vi "interfejs.vi"() -> ()   [LabVIEW 2017]
uses:
  <vilib>/event_ctls.llb/lveventtype.ctl
  <vilib>/Instr/_visa.llb/VISA Configure Serial Port (Instr).vi
  <vilib>/imath/engines/lvmath2/RunTimeEngine/BuiltInFunctions/deg_to_rad/NIMS_deg_to_rad.vi
  <instcachedir>/0/NIMS_deg_to_rad_4A81D684CE8D4DD79924F5AB74D756E1.lvgen/NIMS_deg_to_rad_4A81D684CE8D4DD79924F5AB74D756E1_001.vi
  <vilib>/imath/engines/lvmath2/RunTimeEngine/ArithmeticOperatorToken/NIMS_ArithmeticOperator_multmx-internal.vi
  <instcachedir>/0/NIMS_ArithmeticOperator_multmx-internal_D14B0E8358F948B18FBB33DB0D4CACE1.lvgen/NIMS_ArithmeticOperator_multmx-internal_D14B0E8358F948B18FBB33DB0D4CACE1_004.vi
  <vilib>/imath/engines/lvmath2/RunTimeEngine/ErrorHandling/NIMS_Create Error From Enums.vi
  <vilib>/imath/engines/lvmath2/RunTimeEngine/NodeEndStatement/NIMS_NodeEndStatement_Output.vi
  <instcachedir>/0/NIMS_NodeEndStatement_Output_53EC0D466D134D7ABD903AC30B43404B.lvgen/NIMS_NodeEndStatement_Output_53EC0D466D134D7ABD903AC30B43404B_001.vi
  <vilib>/imath/engines/lvmath2/RunTimeEngine/ErrorHandling/NIMS_Finalize Error.vi
panel:
  out "x/y 5":dbl
  out "x/y 4":dbl
  out "x/y 3":dbl
  out "x/y 2":dbl
  out "x/y":dbl
  in  "SterowanieManipulator":bool
  out "Napięcie akumulatorów":dbl
  out "Temperatura":dbl
  out "Położenie osi skrętnej":u16(knob) scale=0.0..99.0
  out "Zabezpieczenie wyłączenie PWM":string
  out "Kierunek skrętu(1-prawo, 2-lewo)":string
  out "Kierunek jazdy(0-postój, 1-do przodu, 2-do tyłu)":string
  out "readBuffor":string
  out "palec2":i32
  out "pale3":i32
  out "palec4":i32
  out "palec5":i32
  out "X_rekawica":i32
  out "Y_rekawica":i32
  out "palec1":i32
  in  "StartReading":bool
  in  "VISA resource name":refnum<visa-resource-name>
  out "pozycjaSP_manipulator":dbl
  out "pozycjaS1_manipulator":dbl
  out "pozycjaS2_manipulator":dbl
  out "pozycjaS3_manipulator":dbl
  out "Px":dbl
  out "Py":dbl
  out "Pz":dbl
  out "pozycjaS4_manipulator":dbl
  out "pozycjaSn_manipulator":dbl
  in  "UruchomManipulator":bool
  in  "Xn [mm]":dbl=165.0 format="%#_13g"
  in  "X4 [mm]":dbl=205.0 format="%#_13g"
  in  "X3 [mm]":dbl=310.0 format="%#_13g"
  in  "X2[mm]":dbl=400.0 format="%#_13g"
  in  "X1[mm]":dbl=65.0 format="%#_13g"
  in  "Zp [mm]":dbl=465.0 format="%#_13g"
  in  "positionSP [stopnie]":dbl(slide) scale=-85.0..85.0
  in  "positionS1 [stopnie]":dbl(slide)=76.9090909090909 scale=-85.0..85.0
  in  "positionS2 [stopnie]":dbl(slide)=-85.0 scale=-85.0..85.0
  in  "positionS3 [stopnie]":dbl(slide)=-85.0 scale=-85.0..85.0
  in  "positionS4 [stopnie]":dbl(slide)=-52.69090909090909 scale=-85.0..85.0
  in  "positionSn [stopnie]":dbl(slide) scale=-85.0..85.0
  out "ResetPWM_platforma":i16
  out "Brzeczyk_platforma":i16
  out "Swiatla_platforma":i16
  out "BlokadaNapedow_platforma":i16
  out "X_platforma":dbl
  out "Y_platforma":dbl
  out "palce":string
  in  "Typ Sterowania Platforma":bool
  in  "Reset\nzabezpieczenia PWM":bool
  in  "Brzęczyk":bool
  in  "Światła":bool
  in  "Blokada napedów":bool=TRUE
  out "Zadana prędkość":dbl(slide) scale=0.0..99.0
  out "zadany skręt":dbl(slide) scale=0.0..99.0
  out "x1":dbl
  out "y 2":dbl
  in  "Stop":bool
  out "YMysz":dbl
  out "XMysz":dbl
  out "2D Picture":picture
  # "T-rękawica\nF-suwaki"
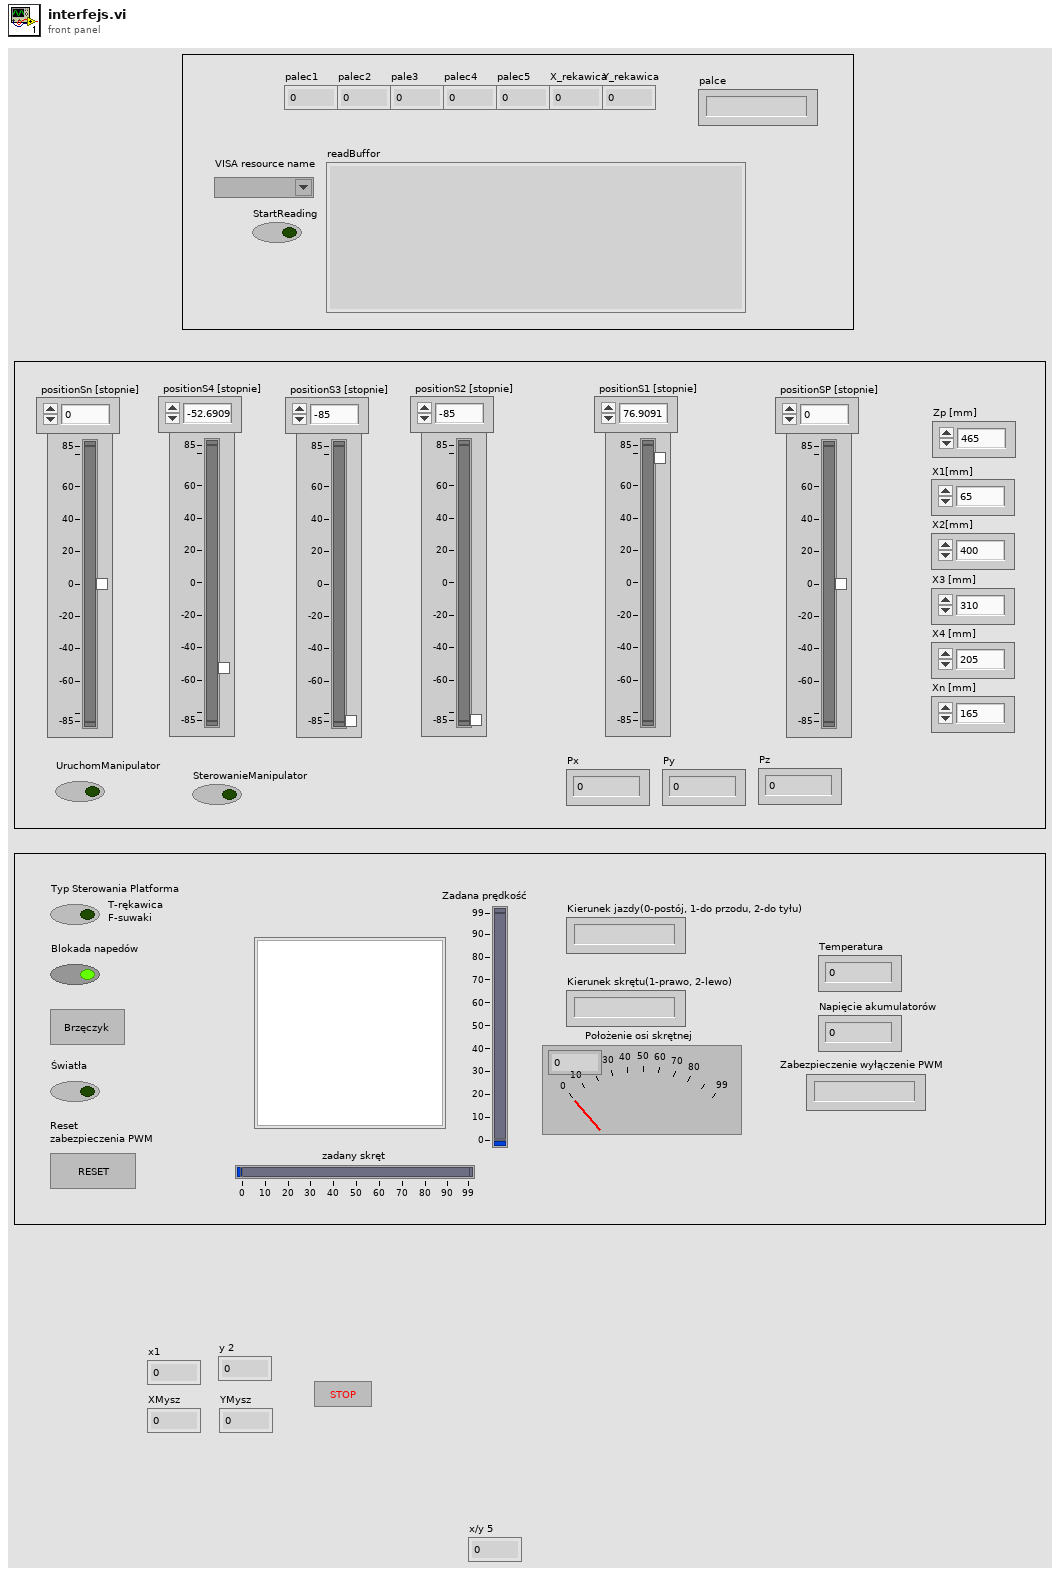
[diagram p1: front panel]
types:
  T1 = enum8{"Enabled", "Disabled", "Disabled and Grayed Out"}
  T2 = typedef "lveventtype.ctl" = enum32{"Null", "Timeout", "Annotation Menu Selection", "Annotation Menu Selection?", "App Instance Close", "App Instance Close?", "Autoscale Range Change", "Bookmark Info Change", "Cell Edit", "Cell Edit?", "Cursor Grab", "Cursor Grab?", "Cursor Menu Selection", "Cursor Menu Selection?", "Cursor Move", "Cursor Release", "Data Change", "Direction Change", "Display State Change", "Drag Ended", "Drag Enter", "Drag Leave", "Drag Over", "Drag Source Update", "Drag Starting", "Drag Starting?", "Drop", "Exec State Change", "Key Down", "Key Down?", "Key Repeat", "Key Repeat?", "Key Up", "Listbox Double Click", "Menu Activation?", "Menu Selection (App)", "Menu Selection? (App)", "Menu Selection (User)", "Mouse Down", "Mouse Down?", "Mouse Enter", "Mouse Leave", "Mouse Move", "Mouse Up", "Mouse Wheel", "NI Security User Change (App)", "Pane Size", "Panel Close", "Panel Close?", "Panel Resize", "Plot Attribute Change", "Scale Range Change", "Shortcut Menu Activation?", "Shortcut Menu Selection (App)", "Shortcut Menu Selection? (App)", "Shortcut Menu Selection (User)", "Tree Double Click", "Tree Drag", "Tree Drag?", "Tree Drop", "Tree Drop?", "Tree Item Close", "Tree Item Close?", "Tree Item Open", "Tree Item Open?", "User Event", "Value Change"}
  T3 = typedef "LVMouseTypeDef.ctl" = cluster{"Mouse Position":cluster{"X":i32, "Y":i32}, "Mouse Modifiers":cluster{"Button Down":bool, "Shift Mod":bool, "Menu Mod":bool, "Option Mod":bool}}
  T4 = typedef "imagedata.ctl" = cluster{"image type":i32, "image depth":i32, "image":u8[], "mask":u8[], "colors":u32[], "Rectangle":cluster{"left":i16, "top":i16, "right":i16, "bottom":i16}}
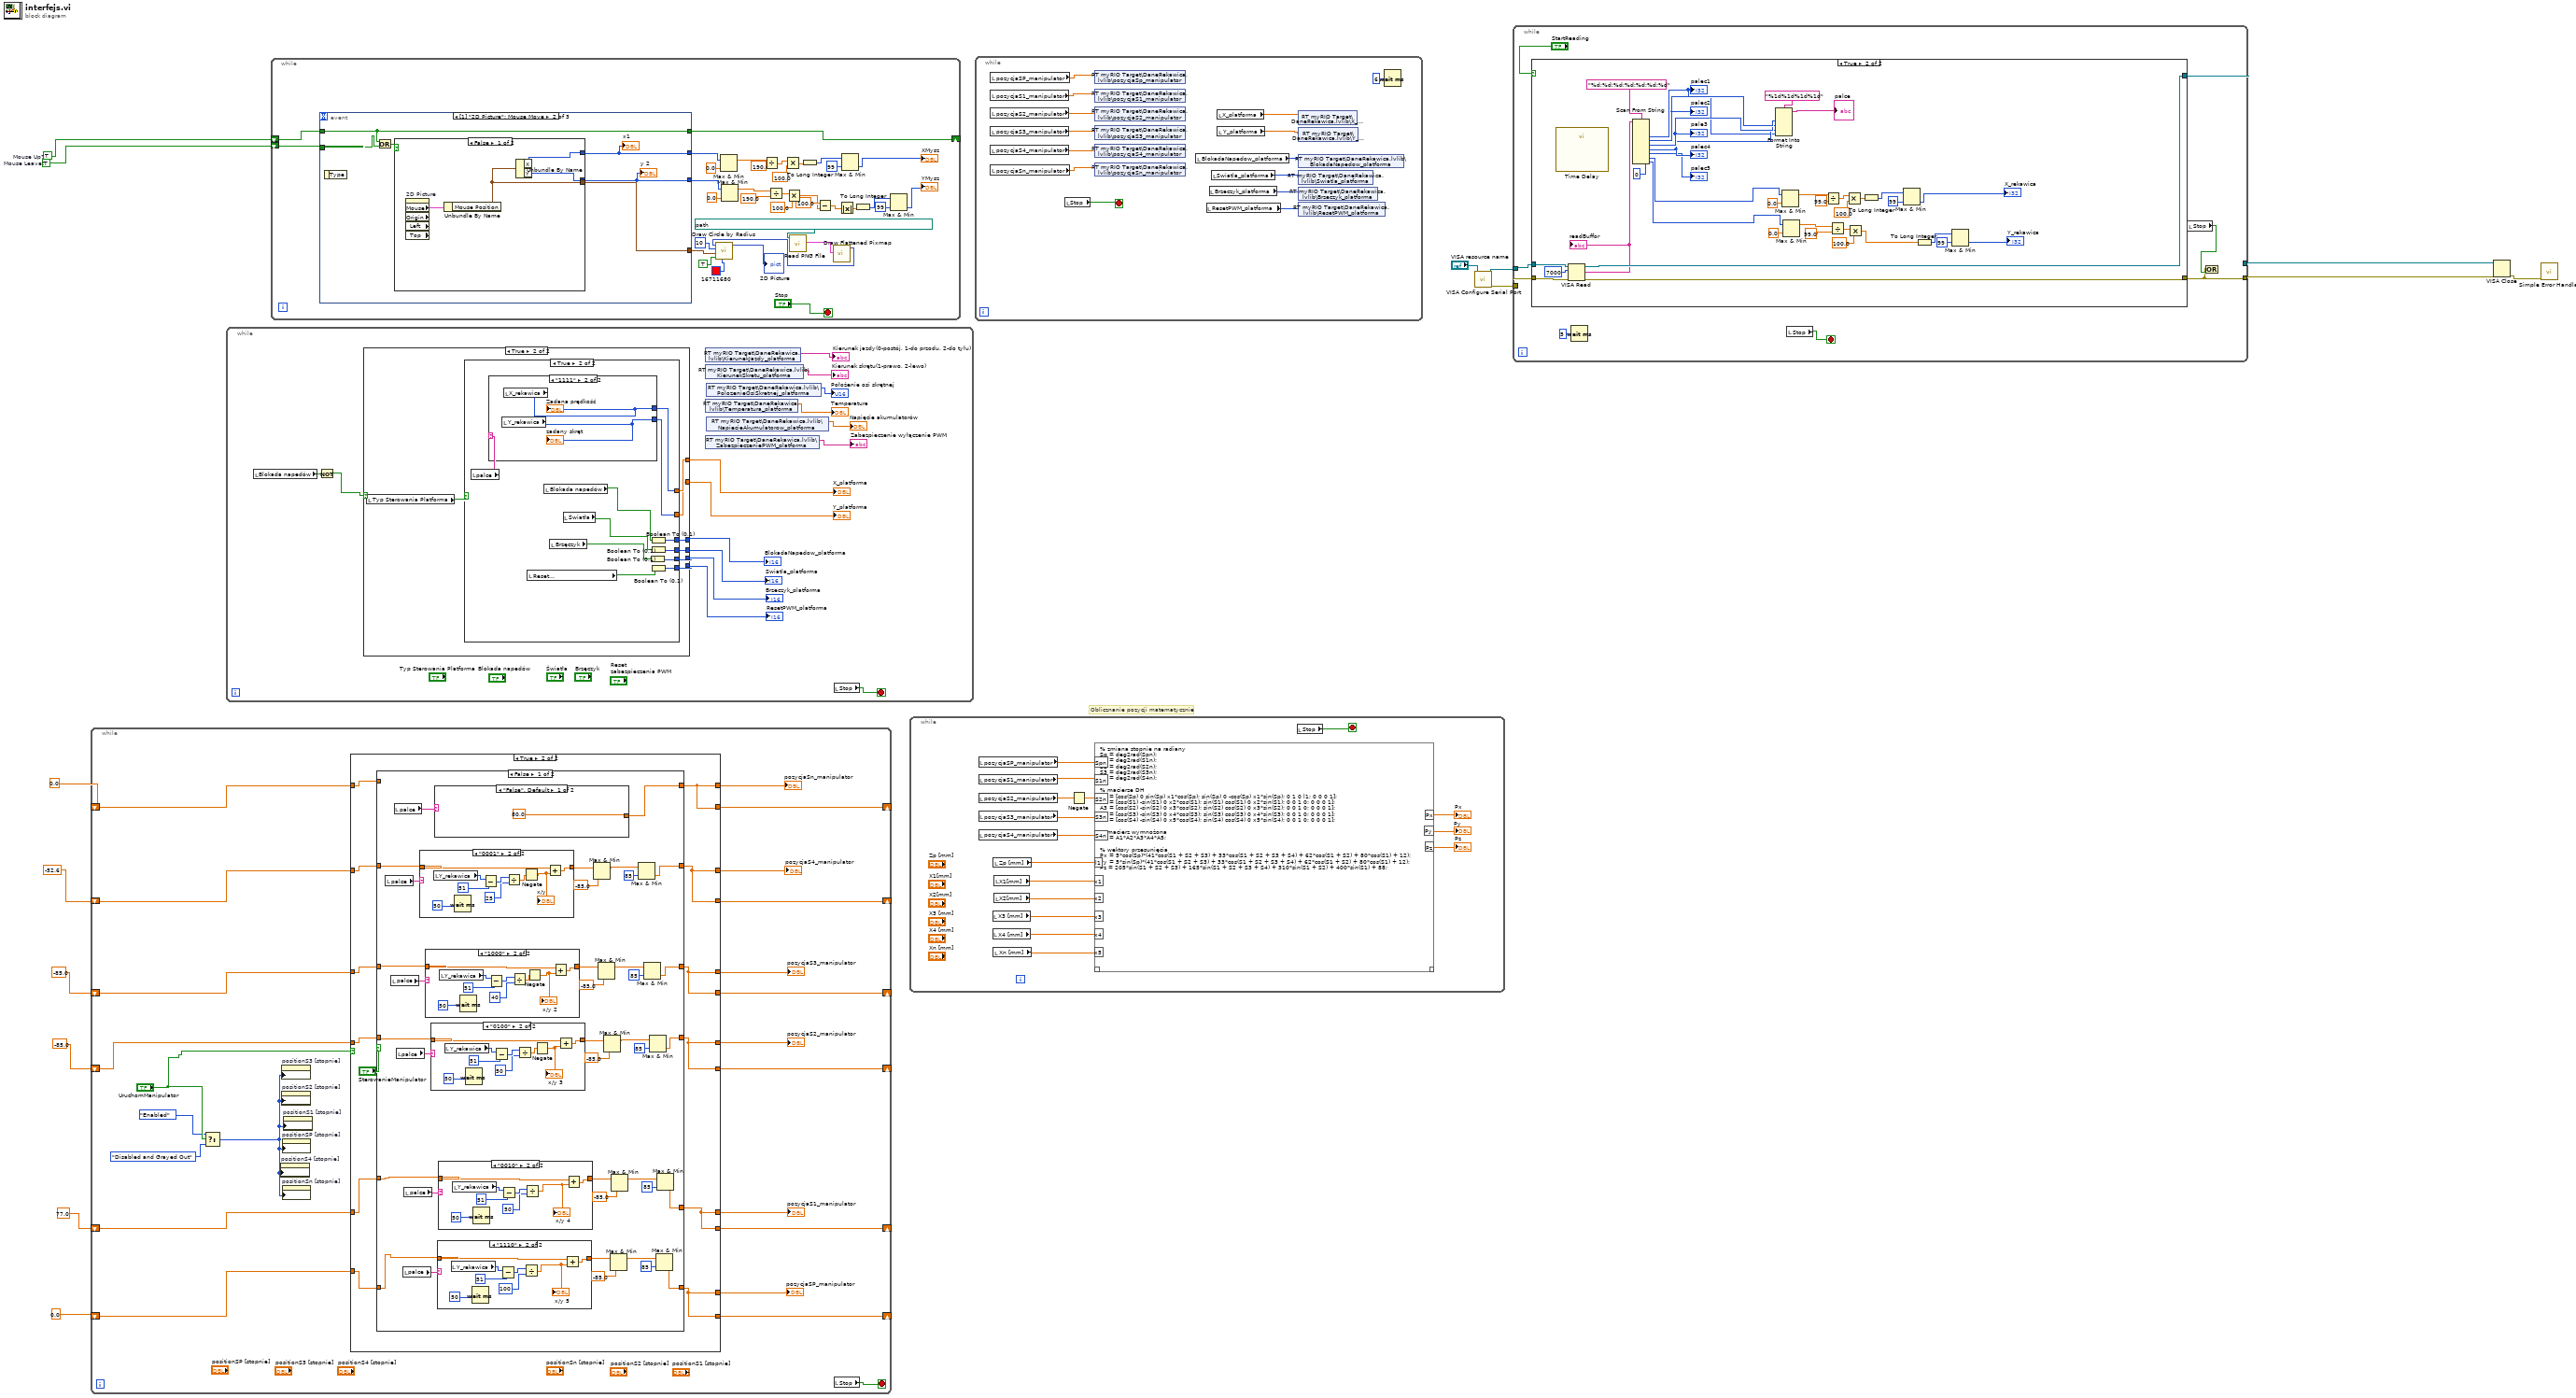
[diagram p0: block diagram]
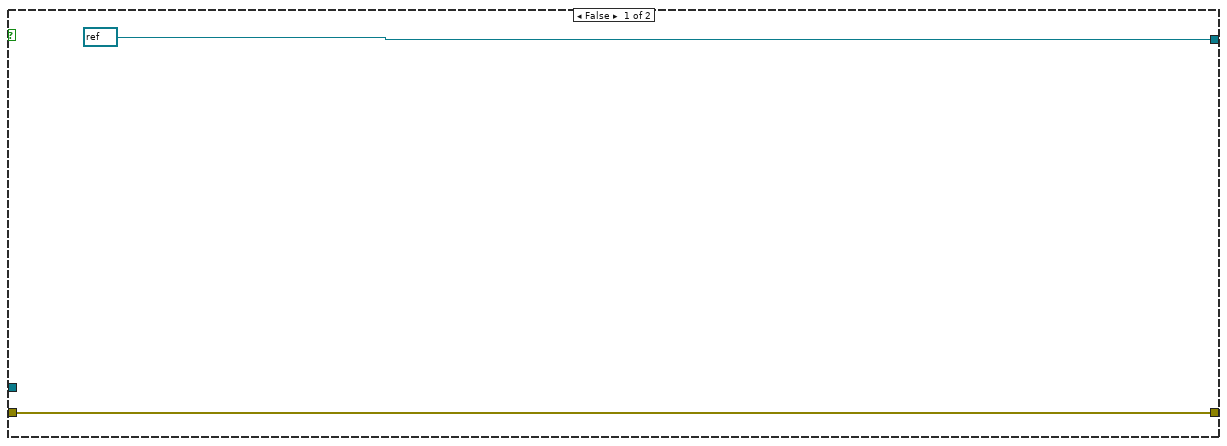
[diagram p2: hidden frame]
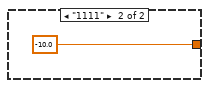
[diagram p4: hidden frame]
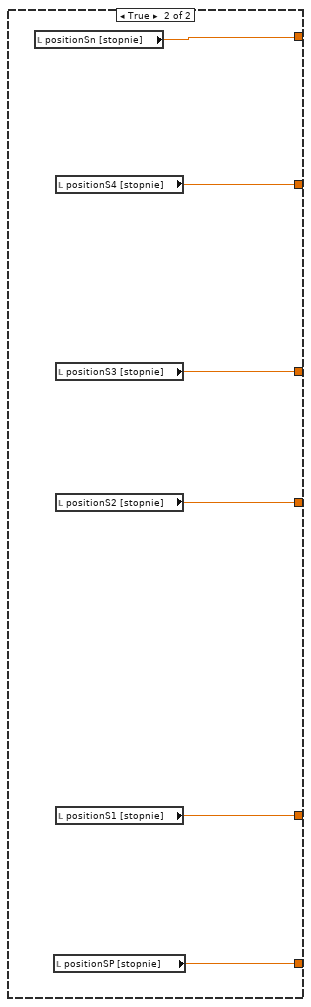
[diagram p10: hidden frame]
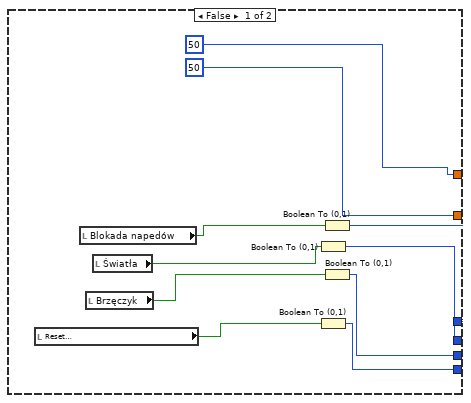
[diagram p11: hidden frame]
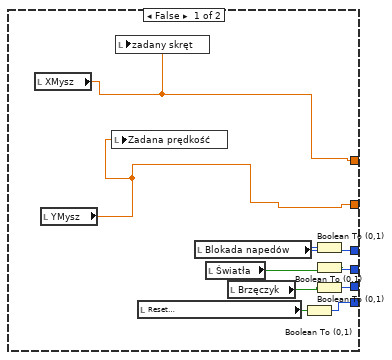
[diagram p12: hidden frame]
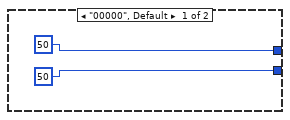
[diagram p13: hidden frame]
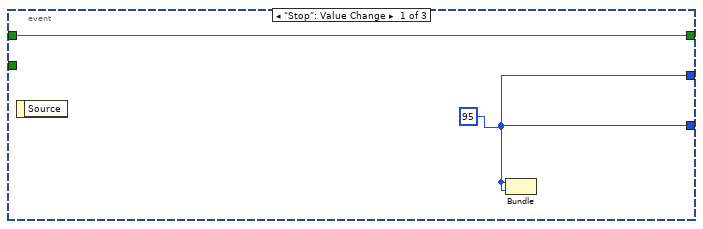
[diagram p14: hidden frame]
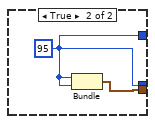
[diagram p15: hidden frame]
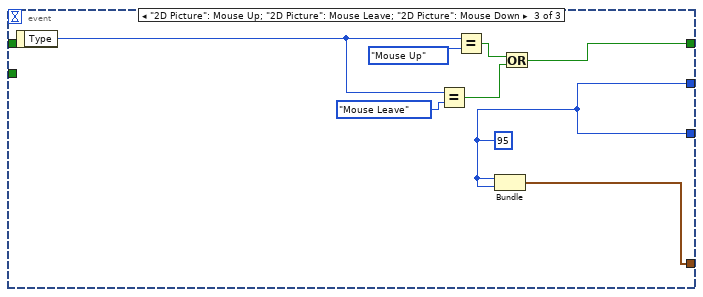
[diagram p16: hidden frame]
diagram:
  w13 = TRUE  # Mouse Leave?
  w14 = TRUE  # Mouse Up?
  # "Oblicznanie pozycji matematycznie"
  n1 = while {
    shift-right: [w24] -> _
    shift-left: 0.0 ("positionSn [stopnie]") -> [w30]
    shift-right: [w23] -> _
    shift-left: -52.6 ("positionS4 [stopnie]") -> [w29]
    shift-right: [w19] -> _
    shift-left: 0.0 ("positionSP [stopnie]") -> [w25]
    shift-right: [w20] -> _
    shift-left: 77.0 ("positionS1 [stopnie]") -> [w26]
    shift-right: [w21] -> _
    shift-left: -85.0 ("positionS2 [stopnie]") -> [w27]
    shift-right: [w22] -> _
    shift-left: -85.0 ("positionS3 [stopnie]") -> [w28]
    stop <- w31 stop-if-true
    n2 = Select(t=T1."Enabled" ("Disabled"), s="UruchomManipulator", f=T1."Disabled and Grayed Out" ("Disabled")) -> (s? t:f=w16:T1)
    n3 = property on="positionS4 [stopnie]" class="Slide (strict)"("DisabledEnum"=w16) -> ()  [unwired: 2 in, 2 out]
    n4 = property on="positionS3 [stopnie]" class="Slide (strict)"("DisabledEnum"=w16) -> ()  [unwired: 2 in, 2 out]
    n5 = property on="positionS2 [stopnie]" class="Slide (strict)"("DisabledEnum"=w16) -> ()  [unwired: 2 in, 2 out]
    n6 = property on="positionSP [stopnie]" class="Slide (strict)"("DisabledEnum"=w16) -> ()  [unwired: 2 in, 2 out]
    n7 = property on="positionSn [stopnie]" class="Slide (strict)"("DisabledEnum"=w16) -> ()  [unwired: 2 in, 2 out]
    n8 = property on="positionS1 [stopnie]" class="Slide (strict)"("DisabledEnum"=w16) -> ()  [unwired: 2 in, 2 out]
    n9 = case shown="True" "UruchomManipulator" {
      tunnel: [w38 w51] -> w37
      tunnel: [w39 w52] -> w32
      tunnel: [w40 w53] -> w33
      tunnel: [w41 w54] -> w34
      tunnel: [w42 w55] -> w35
      tunnel: [w43 w56] -> w36
      tunnel: w30 -> [w43 w48]
      tunnel: w29 -> [w42 w49]
      tunnel: w28 -> [w41 w47]
      tunnel: w27 -> [w40 w46]
      tunnel: w26 -> [w39 w45]
      tunnel: w25 -> [w38 w44]
      tunnel: [w43 w56] -> w24
      tunnel: [w42 w55] -> w23
      tunnel: [w41 w54] -> w22
      tunnel: [w40 w53] -> w21
      tunnel: [w39 w52] -> w20
      tunnel: [w38 w51] -> w19
      frame False {
      }
      frame True {
        n10 = case shown="False" "SterowanieManipulator" {
          tunnel: [w58 w149] -> w56
          tunnel: [w57 w148] -> w55
          tunnel: [w75 w147] -> w54
          tunnel: [w76 w146] -> w53
          tunnel: [w68 w145] -> w52
          tunnel: [w61 w144] -> w51
          tunnel: w49 -> [w93 _]
          tunnel: w48 -> [_ _]
          tunnel: w47 -> [w82 _]
          tunnel: w46 -> [w74 _]
          tunnel: w45 -> [w67 _]
          tunnel: w44 -> [w60 _]
          frame False {
            n11 = local read "palce"() -> (w92:string)
            n12 = local read "palce"() -> (w83:string)
            n13 = local read "palce"() -> (w59:string)
            n14 = local read "palce"() -> (w81:string)
            n15 = local read "palce"() -> (w66:string)
            n16 = local read "palce"() -> (w69:string)
            n17 = case shown="\"0001\"" w92 {
              tunnel: [w134 w143] -> w90
              tunnel: w93 -> [w134 w142]
              frame "0000", Default {
              }
              frame "0001" {
                n18 = local read "Y_rekawica"() -> (w140:i32)
                n19 = Wait (ms)(milliseconds to wait=u32 50) -> ()  [unwired: 1 out]
                n20 = Subtract(x=w140, y=51) -> (x-y=w138:i32)
                n21 = Divide(x=w138, y=25) -> (x/y=w136:dbl)
                n22 = Negate(x=w136) -> (-x=w135:dbl)
                "x/y" <- w135
                n23 = Add(x=w142, y=w135) -> (x+y=w143:dbl)
              }
            }
            n24 = case shown="\"1000\"" w83 {
              tunnel: [w124 w133] -> w85
              tunnel: w82 -> [w124 w132]
              frame "0000", Default {
              }
              frame "1000" {
                n25 = local read "Y_rekawica"() -> (w130:i32)
                n26 = Wait (ms)(milliseconds to wait=u32 50) -> ()  [unwired: 1 out]
                n27 = Subtract(x=w130, y=51) -> (x-y=w128:i32)
                n28 = Divide(x=w128, y=40) -> (x/y=w125:dbl)
                n29 = Negate(x=w125) -> (-x=w126:dbl)
                "x/y 2" <- w126
                n30 = Add(x=w132, y=w126) -> (x+y=w133:dbl)
              }
            }
            n31 = case shown="\"0100\"" w81 {
              tunnel: [w114 w123] -> w79
              tunnel: w74 -> [w114 w122]
              frame "0000", Default {
              }
              frame "0100" {
                n32 = local read "Y_rekawica"() -> (w120:i32)
                n33 = Wait (ms)(milliseconds to wait=u32 50) -> ()  [unwired: 1 out]
                n34 = Subtract(x=w120, y=51) -> (x-y=w118:i32)
                n35 = Divide(x=w118, y=50) -> (x/y=w115:dbl)
                n36 = Negate(x=w115) -> (-x=w116:dbl)
                "x/y 3" <- w116
                n37 = Add(x=w122, y=w116) -> (x+y=w123:dbl)
              }
            }
            n38 = case shown="\"False\", Default" w59 {
              tunnel: [80.0 -10.0] -> w58
              frame "False", Default {
              }
              frame "1111" {
              }
            }
            n39 = case shown="\"1110\"" w66 {
              tunnel: [w96 w104] -> w64
              tunnel: w60 -> [w96 w103]
              frame "0000", Default {
              }
              frame "1110" {
                n40 = local read "Y_rekawica"() -> (w101:i32)
                n41 = Wait (ms)(milliseconds to wait=u32 50) -> ()  [unwired: 1 out]
                n42 = Subtract(x=w101, y=51) -> (x-y=w99:i32)
                n43 = Divide(x=w99, y=100) -> (x/y=w97:dbl)
                "x/y 5" <- w97
                n44 = Add(x=w103, y=w97) -> (x+y=w104:dbl)
              }
            }
            n45 = case shown="\"0010\"" w69 {
              tunnel: [w105 w113] -> w71
              tunnel: w67 -> [w105 w112]
              frame "0000", Default {
              }
              frame "0010" {
                n46 = local read "Y_rekawica"() -> (w110:i32)
                n47 = Wait (ms)(milliseconds to wait=u32 50) -> ()  [unwired: 1 out]
                n48 = Subtract(x=w110, y=51) -> (x-y=w108:i32)
                n49 = Divide(x=w108, y=50) -> (x/y=w106:dbl)
                "x/y 4" <- w106
                n50 = Add(x=w112, y=w106) -> (x+y=w113:dbl)
              }
            }
            n51 = Max & Min(x=w90, y=-85.0) -> (max(x,y)=w88:dbl)  [unwired: 1 out]
            n52 = Max & Min(x=w85, y=-85.0) -> (max(x,y)=w87:dbl)  [unwired: 1 out]
            n53 = Max & Min(x=w79, y=-85.0) -> (max(x,y)=w77:dbl)  [unwired: 1 out]
            n54 = Max & Min(x=w64, y=-85.0) -> (max(x,y)=w62:dbl)  [unwired: 1 out]
            n55 = Max & Min(x=w71, y=-85.0) -> (max(x,y)=w73:dbl)  [unwired: 1 out]
            n56 = Max & Min(x=w88, y=85) -> (min(x,y)=w57:dbl)  [unwired: 1 out]
            n57 = Max & Min(x=w87, y=85) -> (min(x,y)=w75:dbl)  [unwired: 1 out]
            n58 = Max & Min(x=w77, y=85) -> (min(x,y)=w76:dbl)  [unwired: 1 out]
            n59 = Max & Min(x=w62, y=85) -> (min(x,y)=w61:dbl)  [unwired: 1 out]
            n60 = Max & Min(x=w73, y=85) -> (min(x,y)=w68:dbl)  [unwired: 1 out]
          }
          frame True {
            n61 = local read "positionSn [stopnie]"() -> (w149:dbl)
            n62 = local read "positionSP [stopnie]"() -> (w144:dbl)
            n63 = local read "positionS4 [stopnie]"() -> (w148:dbl)
            n64 = local read "positionS3 [stopnie]"() -> (w147:dbl)
            n65 = local read "positionS2 [stopnie]"() -> (w146:dbl)
            n66 = local read "positionS1 [stopnie]"() -> (w145:dbl)
          }
        }
      }
    }
    "pozycjaSn_manipulator" <- w36
    "pozycjaS4_manipulator" <- w35
    "pozycjaS3_manipulator" <- w34
    "pozycjaS2_manipulator" <- w33
    "pozycjaS1_manipulator" <- w32
    "pozycjaSP_manipulator" <- w37
    n67 = local read "Stop"() -> (w31:bool)
  }
  n68 = while {
    stop <- w159 stop-if-true
    n69 = local read "Blokada napedów"() -> (w164:bool)
    n70 = Not(x=w164) -> (.not. x?=w150:bool)
    n71 = case shown="True" w150 {
      tunnel: [w167 w181] -> w163
      tunnel: [w170 w180] -> w162
      tunnel: [w171 w179] -> w161
      tunnel: [w173 w178] -> w160
      tunnel: [50 w176] -> w152
      tunnel: [50 w175] -> w151
      frame False {
        n72 = local read "Reset\nzabezpieczenia PWM"() -> (w174:bool)
        n73 = local read "Blokada napedów"() -> (w168:bool)
        n74 = local read "Brzęczyk"() -> (w172:bool)
        n75 = local read "Światła"() -> (w169:bool)
        n76 = Boolean To (0,1)(Boolean=w169) -> (0, 1=w170:i16)
        n77 = Boolean To (0,1)(Boolean=w174) -> (0, 1=w173:i16)
        n78 = Boolean To (0,1)(Boolean=w168) -> (0, 1=w167:i16)
        n79 = Boolean To (0,1)(Boolean=w172) -> (0, 1=w171:i16)
      }
      frame True {
        n80 = local read "Typ Sterowania Platforma"() -> (w177:bool)
        n81 = case shown="True" w177 {
          tunnel: [w191 w201] -> w181
          tunnel: [w190 w200] -> w180
          tunnel: [w189 w199] -> w179
          tunnel: [w188 w198] -> w178
          tunnel: [w183 w192] -> w176
          tunnel: [w182 w193] -> w175
          frame False {
            n82 = local read "XMysz"() -> (w183:dbl)
            n83 = local read "YMysz"() -> (w182:dbl)
            n84 = local write "Zadana prędkość"(w182) -> ()
            n85 = local write "zadany skręt"(w183) -> ()
            n86 = local read "Reset\nzabezpieczenia PWM"() -> (w184:bool)
            n87 = local read "Blokada napedów"() -> (w187:bool)
            n88 = local read "Światła"() -> (w185:bool)
            n89 = local read "Brzęczyk"() -> (w186:bool)
            n90 = Boolean To (0,1)(Boolean=w184) -> (0, 1=w188:i16)
            n91 = Boolean To (0,1)(Boolean=w187) -> (0, 1=w191:i16)
            n92 = Boolean To (0,1)(Boolean=w185) -> (0, 1=w190:i16)
            n93 = Boolean To (0,1)(Boolean=w186) -> (0, 1=w189:i16)
          }
          frame True {
            n94 = local read "palce"() -> (w202:string)
            n95 = case shown="\"1111\"" w202 {
              tunnel: [50 w206] -> w192
              tunnel: [50 w205] -> w193
              frame "00000", Default {
              }
              frame "1111" {
                n96 = local read "Y_rekawica"() -> (w205:i32)
                "zadany skręt" <- w205
                n97 = local read "X_rekawica"() -> (w206:i32)
                "Zadana prędkość" <- w206
              }
            }
            n98 = local read "Reset\nzabezpieczenia PWM"() -> (w194:bool)
            n99 = local read "Blokada napedów"() -> (w197:bool)
            n100 = local read "Brzęczyk"() -> (w195:bool)
            n101 = local read "Światła"() -> (w196:bool)
            n102 = Boolean To (0,1)(Boolean=w195) -> (0, 1=w199:i16)
            n103 = Boolean To (0,1)(Boolean=w196) -> (0, 1=w200:i16)
            n104 = Boolean To (0,1)(Boolean=w194) -> (0, 1=w198:i16)
            n105 = Boolean To (0,1)(Boolean=w197) -> (0, 1=w201:i16)
          }
        }
      }
    }
    "Y_platforma" <- w151
    "X_platforma" <- w152
    "BlokadaNapedow_platforma" <- w163
    "Swiatla_platforma" <- w162
    "Brzeczyk_platforma" <- w161
    "ResetPWM_platforma" <- w160
    n106 = shared-variable "RT myRIO Target\\DaneRekawica.lvlib\\KierunekJazdy_platforma"() -> (→"Kierunek jazdy(0-postój, 1-do przodu, 2-do tyłu)":string)  [unwired: 1 in, 1 out]
    n107 = shared-variable "RT myRIO Target\\DaneRekawica.lvlib\\ZabezpieczeniePWM_platforma"() -> (→"Zabezpieczenie wyłączenie PWM":string)  [unwired: 1 in, 1 out]
    n108 = shared-variable "RT myRIO Target\\DaneRekawica.lvlib\\KierunekSkretu_platforma"() -> (→"Kierunek skrętu(1-prawo, 2-lewo)":string)  [unwired: 1 in, 1 out]
    n109 = shared-variable "RT myRIO Target\\DaneRekawica.lvlib\\Temperatura_platforma"() -> (→"Temperatura":dbl)  [unwired: 1 in, 1 out]
    n110 = shared-variable "RT myRIO Target\\DaneRekawica.lvlib\\PolozenieOsiSkretnej_platforma"() -> (→"Położenie osi skrętnej":i16)  [unwired: 1 in, 1 out]
    n111 = shared-variable "RT myRIO Target\\DaneRekawica.lvlib\\NapiecieAkumulatorow_platforma"() -> (→"Napięcie akumulatorów":dbl)  [unwired: 1 in, 1 out]
    n112 = local read "Stop"() -> (w159:bool)
  }
  n113 = while {
    shift-right: [w241] -> _
    shift-left: w14 -> [w240]
    shift-left: w13 -> [w235]
    stop <- "Stop" stop-if-true
    n114 = event shown="[1] \"2D Picture\": Mouse Move" {
      selector: _ -> [_ _ _]
      dyn-events: _ -> [_ _ _]
      timeout: _ -> [_ _ _]
      tunnel: [w243 w244 w258] -> w241
      tunnel: w240 -> [w243 w244 _]
      tunnel: [w242 w246 w262] -> w231
      tunnel: [w242 w247 w262] -> w232
      tunnel: w235 -> [_ w248 _]
      tunnel: [_ w245 w256] -> w213
      event "Stop": Value Change {
        w242 = 95
        n115 = event-data() -> ()  [unwired: 1 in, 1 out]
        n116 = Bundle(w242, w242) -> ()  [unwired: 1 in, 1 out]
      }
      event "2D Picture": Mouse Move {
        n117 = event-data() -> ()  [unwired: 1 in, 1 out]
        n118 = Or(x=w244, y=w248) -> (x .or. y?=w249:bool)
        n119 = case shown="False" w249 {
          tunnel: [w252 w255] -> w246
          tunnel: [w251 w255] -> w247
          tunnel: [w250 w254] -> w245
          frame False {
            n120 = property on="2D Picture" class="Pict" props=["Mouse", "Origin", "Left", "Top"]() -> ("Mouse"=w253:T3)  [unwired: 2 in, 5 out]
            n121 = Unbundle By Name(w253) -> ("Mouse Position"=w250:cluster{"X":i32, "Y":i32})
            n122 = Unbundle By Name(w250) -> ("X"=w251:i32, "Y"=w252:i32)
          }
          frame True {
            w255 = 95
            n123 = Bundle(w255, w255) -> (w254:cluster{i32, i32})  [unwired: 1 in]
          }
        }
        "x1" <- w247
        "y 2" <- w246
      }
      event "2D Picture": Mouse Up; "2D Picture": Mouse Leave; "2D Picture": Mouse Down {
        w262 = 95
        n124 = event-data() -> ("Type"=w257:T2)  [unwired: 1 in]
        n125 = Equal?(x=w257, y=lveventtype."Mouse Leave" ("Type")) -> (x = y?=w260:bool)
        n126 = Equal?(x=w257, y=lveventtype."Mouse Up" ("Type")) -> (x = y?=w259:bool)
        n127 = Bundle(w262, w262) -> (w256:cluster{i32, i32})  [unwired: 1 in]
        n128 = Or(x=w259, y=w260) -> (x .or. y?=w258:bool)
      }
    }
    n129 = Max & Min(x=w232, y=0.0) -> (max(x,y)=w230:dbl)  [unwired: 1 out]
    n130 = Max & Min(x=w231, y=0.0) -> (max(x,y)=w229:dbl)  [unwired: 1 out]
    n131 = Divide(x=w230, y=190.0) -> (x/y=w225:dbl)
    n132 = Divide(x=w229, y=190.0) -> (x/y=w226:dbl)
    n133 = Multiply(x=w225, y=100.0) -> (x*y=w222:dbl)
    n134 = Multiply(x=w226, y=100.0) -> (x*y=w219:dbl)
    n135 = call <vilib>:"Read PNG File.vi"("path to PNG file"=path "C:/Users/moko/Desktop/interfejs_użytkownika_MyRIO/sterowaniePlatforma.png") -> ("image data"=w211:T4)  [unwired: 8 in, 2 out]
    n136 = To Long Integer(number=w222) -> (32bit integer=w217:i32)
    n137 = Subtract(x=100.0, y=w219) -> (x-y=w220:dbl)
    n138 = call <vilib>:"Draw Flattened Pixmap.vi"("image data"=w211) -> ("new picture"=w210:picture)  [unwired: 8 in]
    n139 = call <vilib>:"Draw Circle by Radius.vi"("color(black)"=u32 16711680, "fill?(F)"=TRUE, "pixel center"=w213, "radius"=i16 10, "picture"=w210) -> ("new picture"=→"2D Picture":picture)  [unwired: 6 in]
    n140 = Absolute Value(x=w220) -> (abs(x)=w218:dbl)
    n141 = Max & Min(x=w217, y=99) -> (min(x,y)=→"XMysz":i32)  [unwired: 1 out]
    n142 = To Long Integer(number=w218) -> (32bit integer=w214:i32)
    n143 = Max & Min(x=w214, y=99) -> (min(x,y)=→"YMysz":i32)  [unwired: 1 out]
  }
  n144 = while {
    stop <- w278 stop-if-true
    n145 = local read "pozycjaSP_manipulator"() -> (w279:dbl)
    n146 = local read "pozycjaS1_manipulator"() -> (w266:dbl)
    n147 = local read "pozycjaS2_manipulator"() -> (w264:dbl)
    n148 = local read "pozycjaS3_manipulator"() -> (w268:dbl)
    n149 = local read "pozycjaS4_manipulator"() -> (w267:dbl)
    n150 = local read "X3 [mm]"() -> (w275:dbl)
    n151 = local read "X4 [mm]"() -> (w276:dbl)
    n152 = local read "Zp [mm]"() -> (w272:dbl)
    n153 = local read "Xn [mm]"() -> (w277:dbl)
    n154 = local read "X1[mm]"() -> (w273:dbl)
    n155 = local read "X2[mm]"() -> (w274:dbl)
    n156 = Negate(x=w264) -> (-x=w265:dbl)
    n157 = mathscript code="% zmiana stopnie na radiany\nSp = deg2rad(Spn);\nS1 = deg2rad(S1n);\nS2 = deg2rad(S2n);\nS3 = deg2rad(S3n);\nS4 = deg2rad(S4n);\n\n% macierze DH\nA1 = [cos(Sp) 0 sin(Sp) x1*cos(Sp); sin(Sp) 0 -cos(Sp) x1*sin(Sp); 0 1 0 l1; 0 0 0 1];\nA2 = [cos(S1) -sin(S1) 0 x2*cos(S1); sin(S1) cos(S1) 0 x2*sin(S1); 0 0 1 0; 0 0 0 1];\nA3 = [cos(S2) -sin(S2) 0 x3*cos(S2); sin(S2) cos(S2) 0 x3*sin(S2); 0 0 1 0; 0 0 0 1];\nA4 = [cos(S3) -sin(S3) 0 x4*cos(S3); sin(S3) cos(S3) 0 x4*sin(S3); 0 0 1 0; 0 0 0 1];\nA5 = [cos(S4) -sin(S4) 0 x5*cos(S4); sin(S4) cos(S4) 0 x5*sin(S4); 0 0 1 0; 0 0 0 1];\n\n% macierz wymnożona \nT4 = A1*A2*A3*A4*A5;\n\n% wektory przesunięcia\nPx = 5*cos(Sp)*(41*cos(S1 + S2 + S3) + 33*cos(S1 + S2 + S3 + S4) + 62*cos(S1 + S2) + 80*cos(S1) + 12);\nPy = 5*sin(Sp)*(41*cos(S1 + S2 + S3) + 33*cos(S1 + S2 + S3 + S4) + 62*cos(S1 + S2) + 80*cos(S1) + 12);\nPz = 205*sin(S1 + S2 + S3) + 165*sin(S1 + S2 + S3 + S4) + 310*sin(S1 + S2) + 400*sin(S1) + 88;"("Spn"=w279, "S1n"=w266, "S2n"=w265, "S3n"=w268, "S4n"=w267, "l1"=w272, "x1"=w273, "x2"=w274, "x3"=w275, "x4"=w276, "x5"=w277) -> ("Px"=→"Px":dbl, "Py"=→"Py":dbl, "Pz"=→"Pz":dbl)  [unwired: 1 in, 1 out]
    n158 = local read "Stop"() -> (w278:bool)
  }
  n159 = while {
    stop <- w665 stop-if-true
    n160 = local read "pozycjaSP_manipulator"() -> (w664:dbl)
    n161 = local read "pozycjaS1_manipulator"() -> (w663:dbl)
    n162 = local read "pozycjaS2_manipulator"() -> (w662:dbl)
    n163 = local read "pozycjaS3_manipulator"() -> (w661:dbl)
    n164 = local read "pozycjaS4_manipulator"() -> (w660:dbl)
    n165 = local read "pozycjaSn_manipulator"() -> (w659:dbl)
    n166 = local read "Stop"() -> (w665:bool)
    n167 = shared-variable "RT myRIO Target\\DaneRekawica.lvlib\\pozycjaSp_manipulator"(w664) -> ()  [unwired: 1 in, 1 out]
    n168 = shared-variable "RT myRIO Target\\DaneRekawica.lvlib\\pozycjaS1_manipulator"(w663) -> ()  [unwired: 1 in, 1 out]
    n169 = shared-variable "RT myRIO Target\\DaneRekawica.lvlib\\pozycjaS2_manipulator"(w662) -> ()  [unwired: 1 in, 1 out]
    n170 = shared-variable "RT myRIO Target\\DaneRekawica.lvlib\\pozycjaS3_manipulator"(w661) -> ()  [unwired: 1 in, 1 out]
    n171 = shared-variable "RT myRIO Target\\DaneRekawica.lvlib\\pozycjaS4_manipulator"(w660) -> ()  [unwired: 1 in, 1 out]
    n172 = shared-variable "RT myRIO Target\\DaneRekawica.lvlib\\pozycjaSn_manipulator"(w659) -> ()  [unwired: 1 in, 1 out]
    n173 = local read "BlokadaNapedow_platforma"() -> (w669:i16)
    n174 = local read "ResetPWM_platforma"() -> (w672:i16)
    n175 = local read "Brzeczyk_platforma"() -> (w671:i16)
    n176 = local read "Swiatla_platforma"() -> (w670:i16)
    n177 = local read "X_platforma"() -> (w667:dbl)
    n178 = local read "Y_platforma"() -> (w668:dbl)
    n179 = shared-variable "RT myRIO Target\\DaneRekawica.lvlib\\X_platforma"(w667) -> ()  [unwired: 1 in, 1 out]
    n180 = shared-variable "RT myRIO Target\\DaneRekawica.lvlib\\BlokadaNapedow_platforma"(w669) -> ()  [unwired: 1 in, 1 out]
    n181 = shared-variable "RT myRIO Target\\DaneRekawica.lvlib\\Swiatla_platforma"(w670) -> ()  [unwired: 1 in, 1 out]
    n182 = shared-variable "RT myRIO Target\\DaneRekawica.lvlib\\Brzeczyk_platforma"(w671) -> ()  [unwired: 1 in, 1 out]
    n183 = shared-variable "RT myRIO Target\\DaneRekawica.lvlib\\Y_platforma"(w668) -> ()  [unwired: 1 in, 1 out]
    n184 = shared-variable "RT myRIO Target\\DaneRekawica.lvlib\\ResetPWM_platforma"(w672) -> ()  [unwired: 1 in, 1 out]
    n185 = Wait (ms)(milliseconds to wait=u32 6) -> ()  [unwired: 1 out]
  }
  n186 = call-poly "VISA Configure Serial Port"("VISA resource name"="VISA resource name") -> ("VISA resource name out"=w12:refnum<visa-resource-name>, "error out"=w11:errorcluster)  [unwired: 13 in]
  n187 = while {
    tunnel: w12 -> [w676]
    tunnel: w11 -> [w675]
    tunnel: [w674] -> w10
    tunnel: [w673] -> w9
    stop <- w680 stop-if-true
    n188 = case shown="True" "StartReading" {
      tunnel: w675 -> [w682 w717]
      tunnel: w676 -> [_ w716]
      tunnel: [w682 w714] -> w674
      tunnel: [refnum<visa-resource-name> refnum ("VISA resource name out") w711] -> w673
      frame False {
      }
      frame True {
        w712 = 0
        n189 = call "Time Delay"() -> ()  [unwired: 11 in, 1 out]
        n190 = VISA Read(VISA resource name=w716, byte count=u32 7000 ("Read Count"), error in (no error)=w717) -> (VISA resource name out=w711:refnum<visa-resource-name>, read buffer=w689:string, error out=w714:errorcluster)  [unwired: 1 out]
        "readBuffor" <- w689
        n191 = Scan From String(format string="%d;%d;%d;%d;%d;%d;%d", input string=w689, default 1=w712, default 2=w712, default 3=w712, default 4=w712, default 5=w712, default 6=w712, default 7=w712) -> (output 1=w683:i32, output 2=w687:i32, output 3=w686:i32, output 4=w685:i32, output 5=→"palec5":i32, output 6=w691:i32, output 7=w690:i32)  [unwired: 2 in, 3 out]
        "palec2" <- w687
        "pale3" <- w686
        "palec4" <- w685
        "palec1" <- w683
        n192 = Format Into String(format string="%1d%1d%1d%1d", w687, w686, w685, w683) -> (resulting string=→"palce":string)  [unwired: 2 in, 1 out]
        n193 = Max & Min(x=w691, y=0.0) -> (max(x,y)=w706:dbl)  [unwired: 1 out]
        n194 = Max & Min(x=w690, y=0.0) -> (max(x,y)=w705:dbl)  [unwired: 1 out]
        n195 = Divide(x=w706, y=99.0) -> (x/y=w701:dbl)
        n196 = Divide(x=w705, y=99.0) -> (x/y=w702:dbl)
        n197 = Multiply(x=w701, y=100.0) -> (x*y=w698:dbl)
        n198 = Multiply(x=w702, y=100.0) -> (x*y=w688:dbl)
        n199 = To Long Integer(number=w698) -> (32bit integer=w697:i32)
        n200 = Max & Min(x=w697, y=99) -> (min(x,y)=→"X_rekawica":i32)  [unwired: 1 out]
        n201 = To Long Integer(number=w688) -> (32bit integer=w694:i32)
        n202 = Max & Min(x=w694, y=99) -> (min(x,y)=→"Y_rekawica":i32)  [unwired: 1 out]
      }
    }
    n203 = Wait (ms)(milliseconds to wait=u32 5) -> ()  [unwired: 1 out]
    n204 = local read "Stop"() -> (w680:bool)
    n205 = local read "Stop"() -> (w678:bool)
    n206 = Or(x=w674, y=w678) -> ()  [unwired: 1 out]
  }
  n207 = VISA Close(VISA resource name=w9, error in (no error)=w10) -> (error out=w8:errorcluster)
  n208 = call <vilib>:"Simple Error Handler.vi"("error in (no error)"=w8) -> ()  [unwired: 4 in, 5 out]
